vi "Segment Creater.vi"(6 "Time Period":i8, 7 "Max profiles":T1, 8 "VelocityAtEnd":dbl, 9 "PositionAtEnd":dbl, 10 "StartTime":dbl, 11 "TimePeriod":dbl) -> (0 "TimeAtEnd":dbl, 3 "TimeSegment":T2)   [LabVIEW 2014]
uses:
  TimeSegment.ctl
  Max profiles.ctl
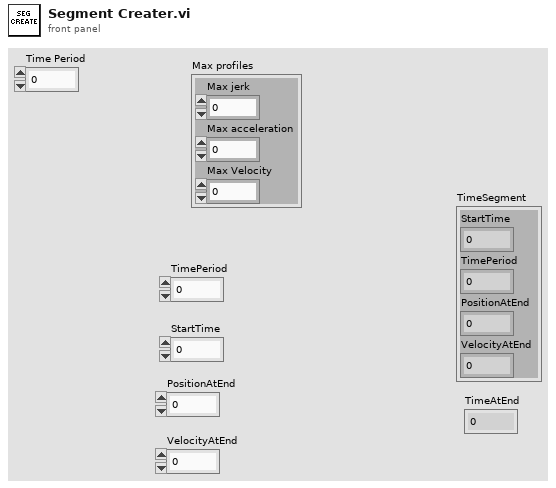
[diagram p1: front panel]
types:
  T1 = typedef "Max profiles.ctl" = cluster{"Max jerk":dbl, "Max acceleration":dbl, "Max Velocity":dbl}
  T2 = typedef "TimeSegment.ctl" = cluster{"StartTime":dbl, "TimePeriod":dbl, "PositionAtEnd":dbl, "VelocityAtEnd":dbl}
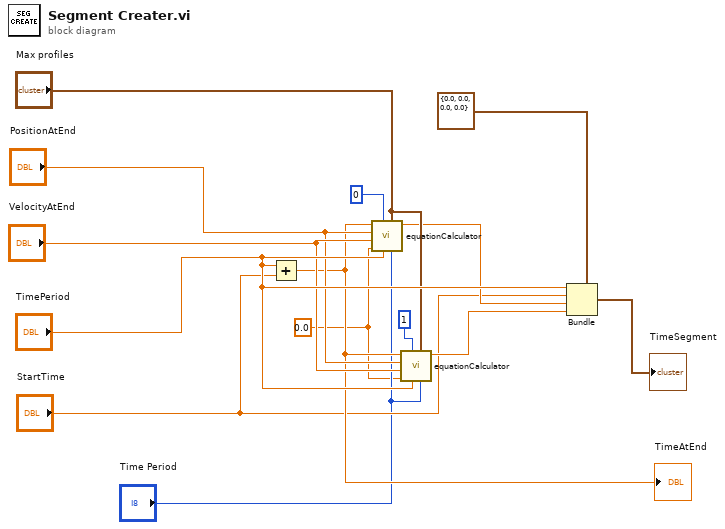
[diagram p0: block diagram]
diagram:
  w1 = 0.0 ("aInital (only needed for T0)")
  n1 = Add(x="TimePeriod", y="StartTime") -> (x+y=w9:dbl)
  "TimeAtEnd" <- w9
  n2 = call "equationCalculator.vi"("Time Period"="Time Period", "Max profiles"="Max profiles", "startOfTimePeriod"="TimePeriod", "derivitave"=i8 0, "aInital (only needed for T0)"=w1, "vInital"="VelocityAtEnd", "xInital"="PositionAtEnd", "currentTime"=w9) -> ("output variable"=w6:dbl)  [unwired: 3 in]
  n3 = call "equationCalculator.vi"("Time Period"="Time Period", "Max profiles"="Max profiles", "startOfTimePeriod"="TimePeriod", "derivitave"=i8 1 ("Time Period"), "aInital (only needed for T0)"=w1, "vInital"="VelocityAtEnd", "xInital"="PositionAtEnd", "currentTime"=w9) -> ("output variable"=w13:dbl)  [unwired: 3 in]
  n4 = Bundle(cluster=T2 {"StartTime"=0.0, "TimePeriod"=0.0, "PositionAtEnd"=0.0, "VelocityAtEnd"=0.0} ("TimeSegment"), "StartTime"="TimePeriod", "TimePeriod"="StartTime", "PositionAtEnd"=w6, "VelocityAtEnd"=w13) -> (→"TimeSegment":T2)
